vi "QSM - Initialize.vi"(8 "Error In":errorcluster, 11 "Invalid Option":T1=enum."Ignore") -> (0 "Error Out":errorcluster, 4 "QSM":T2={"Invalid Option"=enum."Ignore", "QSM"=refnum})   [LabVIEW 2014]
doc: "This is the initialization VI. It allows you to configure how to handle invalid state names\n\nDataEtc Copyright (c) 2013"
uses:
  TypeDef/QSM - STYP.ctl
  TypeDef/Invalid Option - STYP.ctl
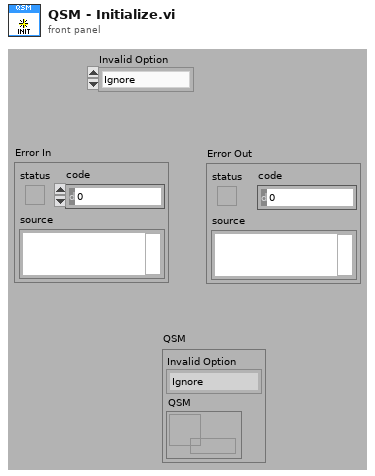
[diagram p1: front panel]
types:
  T1 = typedef "Invalid Option - STYP.ctl" = enum16{"Dialog", "Error", "Ignore"}
  T2 = typedef "QSM - STYP.ctl" = cluster{"Invalid Option":T1, "QSM":refnum<queue>}
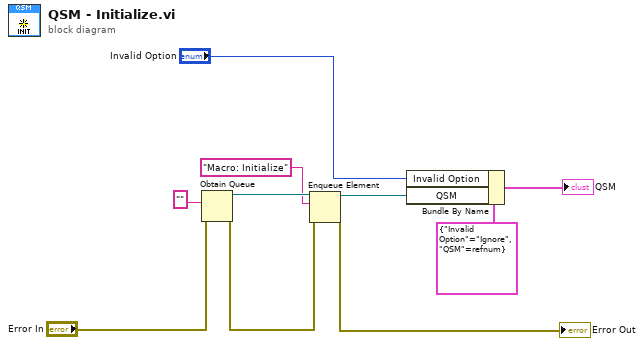
[diagram p0: block diagram]
diagram:
  n1 = Obtain Queue(element data type="", error in (no error)="Error In") -> (queue out=w9:refnum<queue>, error out=w8:errorcluster)  [unwired: 2 in, 2 out]
  n2 = Enqueue Element(queue=w9, element="Macro: Initialize", error in (no error)=w8) -> (queue out=w6:refnum<queue>, error out=→"Error Out":errorcluster)  [unwired: 2 out]
  n3 = Bundle By Name(cluster=T2 {"Invalid Option"=enum."Ignore", "QSM"=refnum} ("ASC QSM"), "Invalid Option"="Invalid Option", "QSM"=w6) -> (→"QSM":T2)
